vi "Choose Annotation.vi"(8 "Error In":errorcluster) -> (0 "Error Out":errorcluster, 3 "String chosen":string)   [LabVIEW 2017]
uses:
  Controls/Annotation SONONet.ctl
panel:
  in  "Cancel Button":bool
  in  "OK Button":bool
  in  "Annotation":T1=13 items=["Brain (cb.)", "Brain (tv.)", "Lips", "Abdominal", "Kidneys", "Femur", "Spine (sag.)", "Spine (cor.)", "4CH", "3VV", "RVOT", "LVOT", "Profile", "Background"]
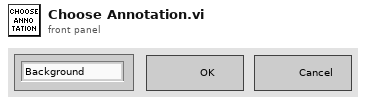
[diagram p1: front panel]
types:
  T1 = typedef "Annotation SONONet.ctl" = u16
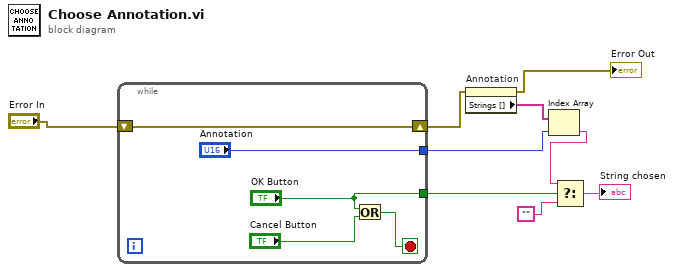
[diagram p0: block diagram]
diagram:
  n1 = while {
    tunnel: ["Annotation"] -> w8
    tunnel: ["OK Button"] -> w7
    shift-right: [w10] -> w2
    shift-left: "Error In" -> [w10]
    stop <- w12 stop-if-true
    n2 = Or(x="OK Button", y="Cancel Button") -> (x .or. y?=w12:bool)
  }
  n3 = property on="Annotation" class="Ring (strict)"(error in=w2) -> (error out=→"Error Out":errorcluster, "Strings []"=w9:string[])  [unwired: 1 in, 1 out]
  n4 = Index Array(array=w9, index=w8) -> (element=w6:string)
  n5 = Select(t=w6, s=w7, f="") -> (s? t:f=→"String chosen":string)
